vi "Save As Sif.vi"(8 "error in (no error)":errorcluster, 11 "CCDCamera in":refnum<class "CCDCamera.lvclass">) -> (0 "error out":errorcluster, 3 "CCDCamera out":refnum<class "CCDCamera.lvclass">)   [LabVIEW 2018, in "CCDCamera.lvclass"]
doc: "Este VI salva a última imagem obtida pelo CCD no format Sif."
uses:
  CCDCamera.lvclass
  CCDCamera.lvclass/CCDCamera.ctl
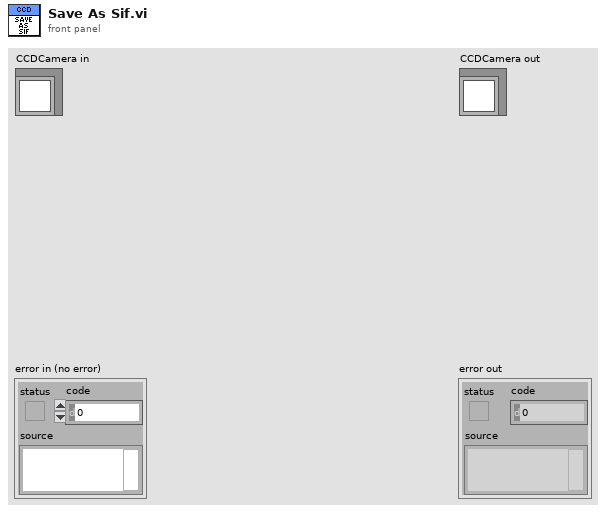
[diagram p1: front panel]
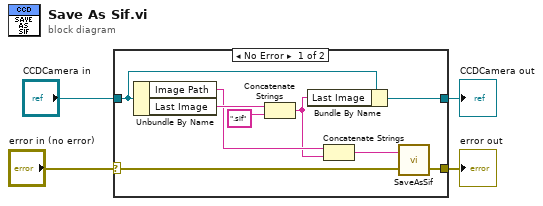
[diagram p0: block diagram]
diagram:
  n1 = case shown="No Error" "error in (no error)" {
    selector: "error in (no error)" -> [w13 w15]
    tunnel: [w12 w15] -> w3
    tunnel: [w10 w14] -> w1
    tunnel: "CCDCamera in" -> [w9 w14]
    frame No Error {
      n2 = Unbundle By Name(w9) -> ("Image Path"=w6:string, "Last Image"=w8:string)
      n3 = Concatenate Strings(w8, ".sif" ("string")) -> (w5:string)
      n4 = Bundle By Name(cluster=w9, "Last Image"=w5) -> (w10:refnum<class "CCDCamera.lvclass">)
      n5 = Concatenate Strings(w6, w5) -> (w7:string)
      n6 = call <userlib>:"SaveAsSif.vi"("error in (no error)"=w13, "path"=w7) -> ("error out"=w12:errorcluster)  [unwired: 1 out]
    }
    frame Error {
    }
  }
  "error out" <- w3
  "CCDCamera out" <- w1
